vi "Find Owned Test Methods.vi"(8 "error in (no error)":errorcluster, 10 "Test Methods In":map{string, path}(c390), 11 "LVClassLibrary in":refnum<vi>) -> (0 "error out":errorcluster, 2 "Test Methods Out":map{string, path}(c390), 3 "LVClassLibrary out":refnum<vi>)   [LabVIEW 2020, in "Test Finder.lvclass"]
uses:
  Test Finder.lvclass
  Test Finder.lvclass/Test Finder.ctl
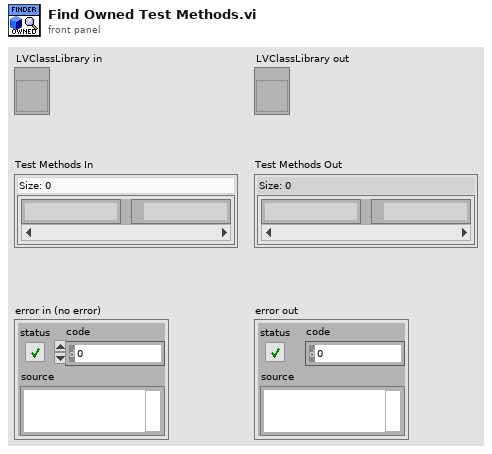
[diagram p1: front panel]
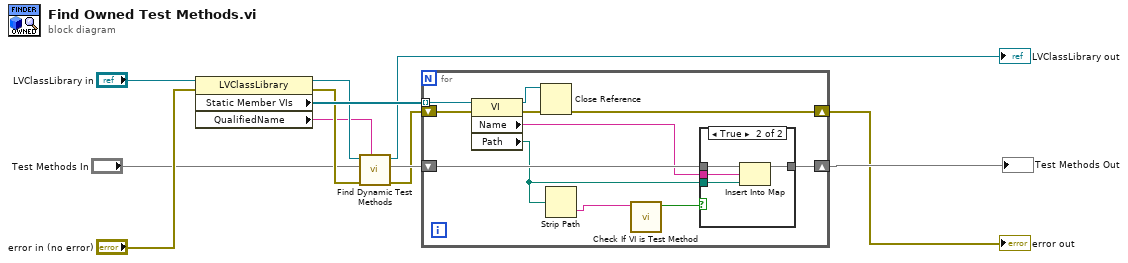
[diagram p0: block diagram]
diagram:
  n1 = property class="LVClassLibrary"(reference="LVClassLibrary in", error in="error in (no error)") -> (reference out=w7:refnum<vi>, error out=w5:errorcluster, "Static Member VIs"=w10:refnum<vi>[], "QualifiedName"=w1:string)
  n2 = call "Find Dynamic Test Methods.vi"("Test Case class name"=w1, "error in (no error)"=w5, "Test Methods In"="Test Methods In", "LVClassLibrary in"=w7) -> ("error out"=w2:errorcluster, "Test Methods Out"=w3:map{string, path}, "LVClassLibrary out"=→"LVClassLibrary out":refnum<vi>)  [unwired: 5 in]
  n3 = for {
    tunnel: w10 -> [w23] mode=indexing
    shift-right: [w19] -> w8
    shift-left: w2 -> [w22]
    shift-right: [w17] -> w9
    shift-left: w3 -> [w18]
    n4 = property class="VI"(reference=w23, error in=w22) -> (reference out=w20:refnum<vi>, error out=w21:errorcluster, "Name"=w16:string, "Path"=w14:path)
    n5 = Close Reference(reference=w20, error in (no error)=w21) -> (error out=w19:errorcluster)
    n6 = Strip Path(path=w14) -> (name=w13:string)  [unwired: 1 out]
    n7 = call "Check If VI is Test Method.vi"("VI Name"=w13) -> ("Is Test Method?"=w15:bool)  [unwired: 9 in, 1 out]
    n8 = case shown="True" w15 {
      tunnel: w18 -> [w24 w28]
      tunnel: w14 -> [_ w27]
      tunnel: [w24 w26] -> w17
      tunnel: w16 -> [_ w25]
      frame False {
      }
      frame True {
        n9 = Insert Into Map(map in=w28, key=w25, value=w27) -> (map out=w26:map{string, path})  [unwired: 2 out]
      }
    }
  }
  "error out" <- w8
  "Test Methods Out" <- w9
